vi "FTW-JSON-Interpret-Core.vi"(5 "JSON String":string, 7 "JSON Parent":T1, 9 "Starting Offset":i32, 11 "error in":errorcluster) -> (4 "Data Name":string, 6 "JSON Part":T1, 8 "Container":variant, 10 "Offset after Match":i32, 14 "Found Match?":bool, 15 "error out":errorcluster)   [LabVIEW 2015]
uses:
  FTW-JSON-Part.ctl
panel:
  out "Match":string
  # "Inputs"
  # "Outputs"
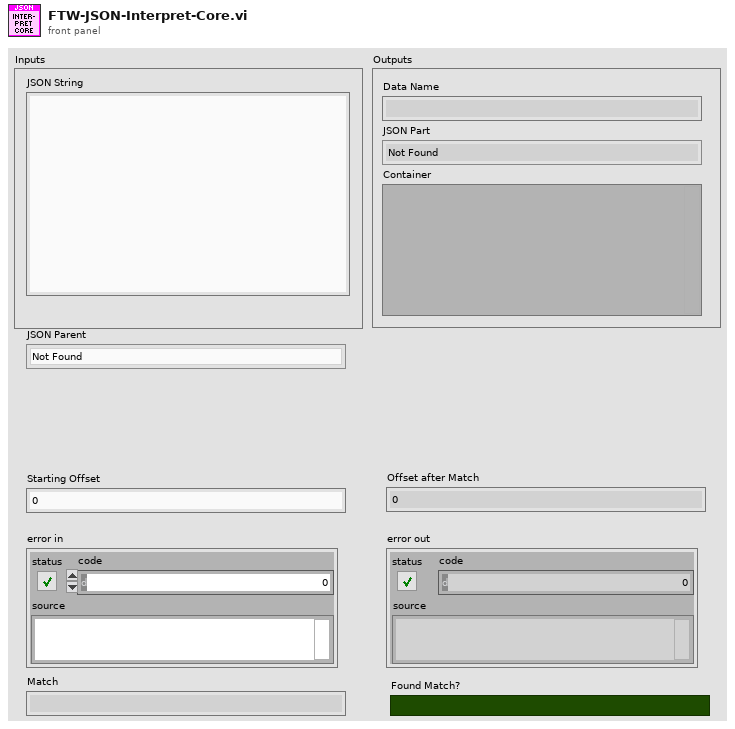
[diagram p1: front panel]
types:
  T1 = typedef "FTW-JSON-Part.ctl" = enum8{"Not Found", "Object", "Object Inner", "Array", "Array Inner", "String", "Number", "Boolean", "null"}
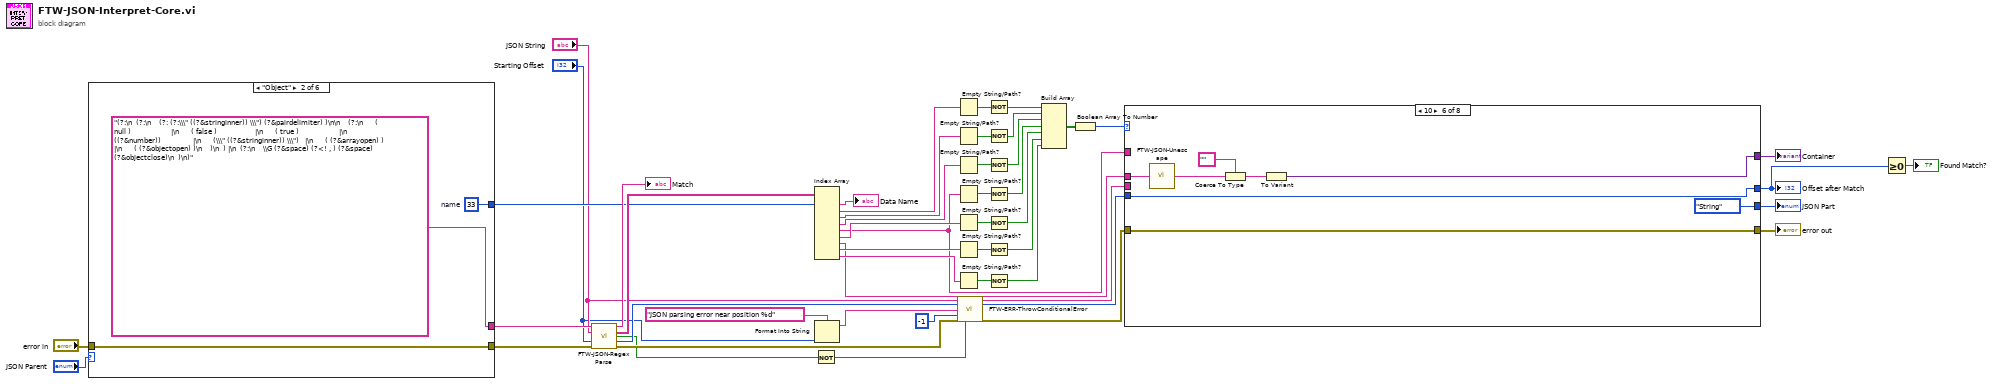
[diagram p0: block diagram]
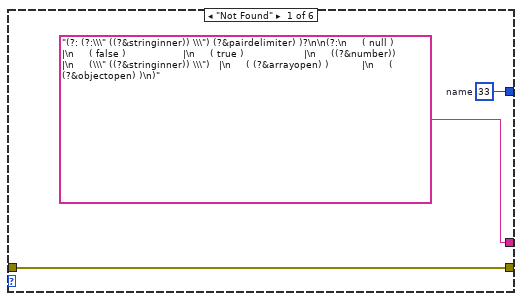
[diagram p2: hidden frame]
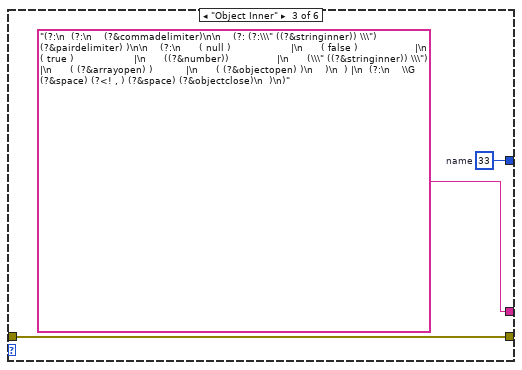
[diagram p3: hidden frame]
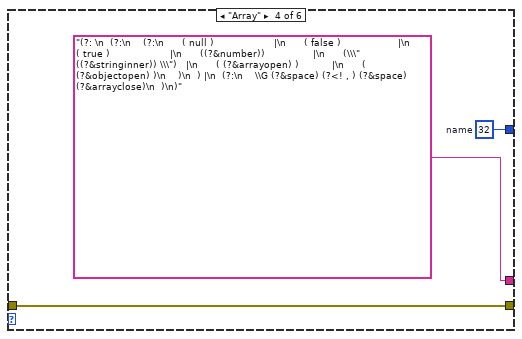
[diagram p4: hidden frame]
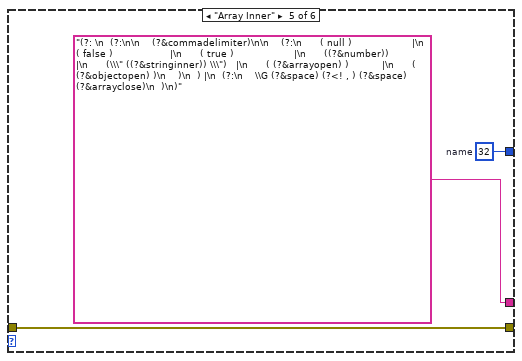
[diagram p5: hidden frame]
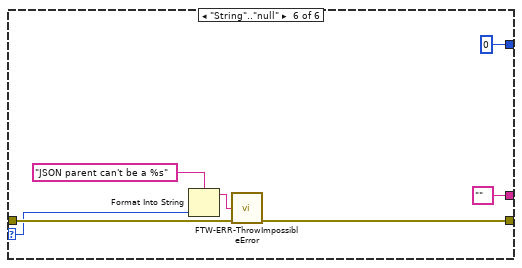
[diagram p6: hidden frame]
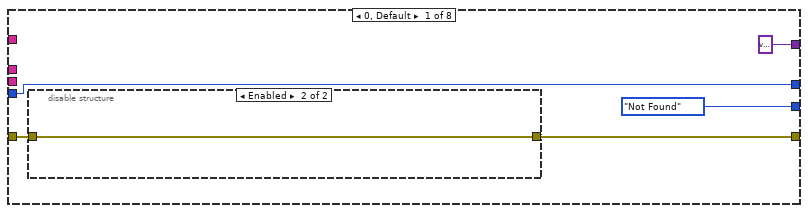
[diagram p7: hidden frame]
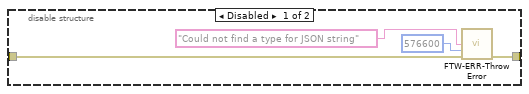
[diagram p8: hidden frame]
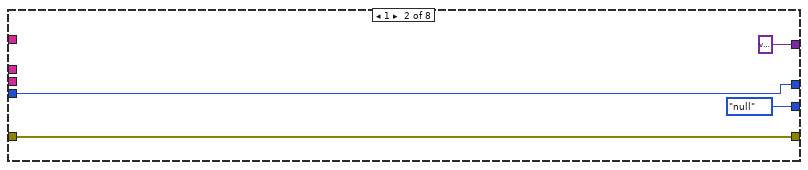
[diagram p9: hidden frame]
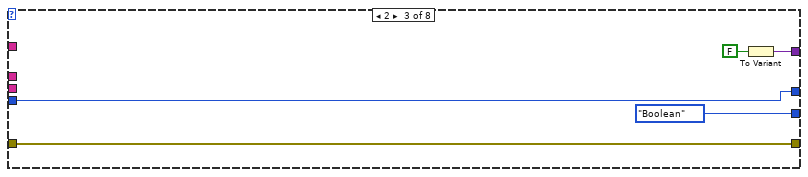
[diagram p10: hidden frame]
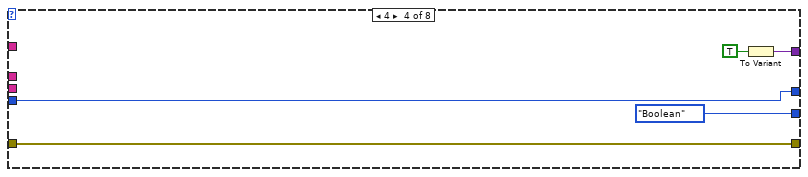
[diagram p11: hidden frame]
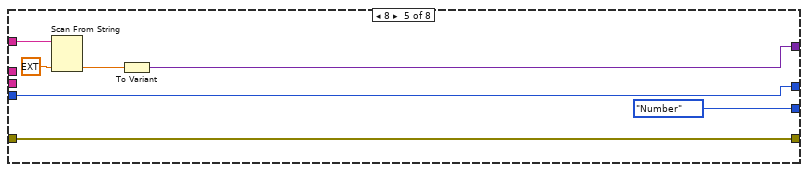
[diagram p12: hidden frame]
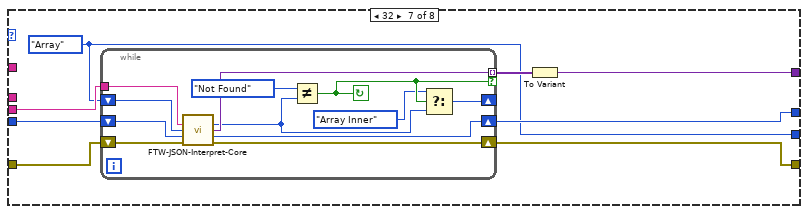
[diagram p13: hidden frame]
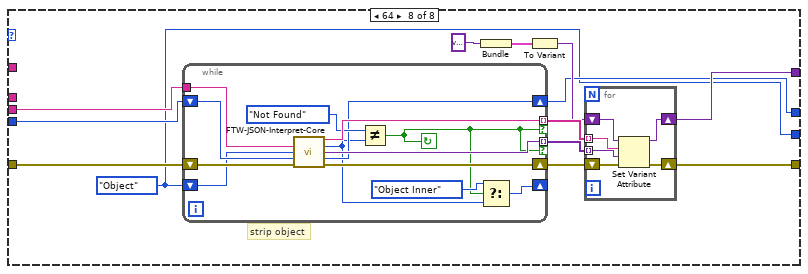
[diagram p14: hidden frame]
diagram:
  n1 = case shown="\"Object\"" "JSON Parent" {
    selector: "JSON Parent" -> [_ _ _ _ _ w66]
    tunnel: ["(?: (?:\\\" ((?&stringinner)) \\\") (?&pairdelimiter) )?\n\n(?:\n     ( null )                    |\n     ( false )                   |\n     ( true )                    |\n     ((?&number))                |\n     (\\\" ((?&stringinner)) \\\")   |\n     ( (?&arrayopen) )           |\n     ( (?&objectopen) )\n)" "(?:\n  (?:\n    (?: (?:\\\" ((?&stringinner)) \\\") (?&pairdelimiter) )\n\n    (?:\n      ( null )                    |\n      ( false )                   |\n      ( true )                    |\n      ((?&number))                |\n      (\\\" ((?&stringinner)) \\\")   |\n      ( (?&arrayopen) )           |\n      ( (?&objectopen) )\n    )\n  ) |\n  (?:\n    \\G (?&space) (?<! , ) (?&space) (?&objectclose)\n  )\n)" "(?:\n  (?:\n    (?&commadelimiter)\n\n    (?: (?:\\\" ((?&stringinner)) \\\") (?&pairdelimiter) )\n\n    (?:\n      ( null )                    |\n      ( false )                   |\n      ( true )                    |\n      ((?&number))                |\n      (\\\" ((?&stringinner)) \\\")   |\n      ( (?&arrayopen) )           |\n      ( (?&objectopen) )\n    )\n  ) |\n  (?:\n    \\G (?&space) (?<! , ) (?&space) (?&objectclose)\n  )\n)" "(?: \n  (?:\n    (?:\n      ( null )                    |\n      ( false )                   |\n      ( true )                    |\n      ((?&number))                |\n      (\\\" ((?&stringinner)) \\\")   |\n      ( (?&arrayopen) )           |\n      ( (?&objectopen) )\n    )\n  ) |\n  (?:\n    \\G (?&space) (?<! , ) (?&space) (?&arrayclose)\n  )\n)" "(?: \n  (?:\n\n    (?&commadelimiter)\n\n    (?:\n      ( null )                    |\n      ( false )                   |\n      ( true )                    |\n      ((?&number))                |\n      (\\\" ((?&stringinner)) \\\")   |\n      ( (?&arrayopen) )           |\n      ( (?&objectopen) )\n    )\n  ) |\n  (?:\n    \\G (?&space) (?<! , ) (?&space) (?&arrayclose)\n  )\n)" "" ("empty string")] -> w13
    tunnel: [w49 w52 w55 w58 w61 w68] -> w20
    tunnel: "error in" -> [w49 w52 w55 w58 w61 w69]
    tunnel: [w48 w51 w54 w57 w60 0] -> w18
    frame "Not Found" {
      w48 = 33  # name
    }
    frame "Object" {
      w51 = 33  # name
    }
    frame "Object Inner" {
      w54 = 33  # name
    }
    frame "Array" {
      w57 = 32  # name
    }
    frame "Array Inner" {
      w60 = 32  # name
    }
    frame "String".."null" {
      n2 = Format Into String(format string="JSON parent can't be a %s" ("Reason this error should never happen"), w66) -> (resulting string=w65:string)  [unwired: 2 in, 1 out]
      n3 = call "FTW-ERR-ThrowImpossibleError.vi"("Reason this error should never happen"=w65, "error in"=w69) -> ("error out"=w68:errorcluster)  [unwired: 13 in]
    }
  }
  n4 = call "FTW-JSON-RegexParse.vi"("Regular Expression using JSON subroutines"=w13, "Input String"="JSON String", "Starting Offset"="Starting Offset", "error in"=w20) -> ("Match"=→"Match":string, "Submatches"=w40:string[], "Found Match?"=w8:bool, "Offset after Match"=w12:i32, "error out"=w43:errorcluster)  [unwired: 7 in]
  n5 = Not(x=w8) -> (.not. x?=w7:bool)
  n6 = Index Array(array=w40, index #1=w18) -> (element #1=→"Data Name":string, element #2=w41:string, element #3=w34:string, element #4=w28:string, element #5=w11:string, element #6=w15:string, element #7=w14:string, element #8=w17:string, element #9=w16:string)  [unwired: 8 in]
  n7 = Format Into String(format string="JSON parsing error near position %d", "Starting Offset") -> (resulting string=w4:string)  [unwired: 2 in, 1 out]
  n8 = Empty String/Path?(string/path=w41) -> (empty?=w39:bool)
  n9 = Empty String/Path?(string/path=w34) -> (empty?=w35:bool)
  n10 = Empty String/Path?(string/path=w28) -> (empty?=w32:bool)
  n11 = Empty String/Path?(string/path=w11) -> (empty?=w31:bool)
  n12 = Empty String/Path?(string/path=w15) -> (empty?=w27:bool)
  n13 = Empty String/Path?(string/path=w17) -> (empty?=w24:bool)
  n14 = Empty String/Path?(string/path=w16) -> (empty?=w25:bool)
  n15 = call "FTW-ERR-ThrowConditionalError.vi"("Error Message"=w4, "Error Code"=-1, "error in"=w43, "Throw Error?"=w7) -> ("error out"=w9:errorcluster)  [unwired: 11 in]
  n16 = Not(x=w39) -> (.not. x?=w38:bool)
  n17 = Not(x=w35) -> (.not. x?=w33:bool)
  n18 = Not(x=w32) -> (.not. x?=w30:bool)
  n19 = Not(x=w31) -> (.not. x?=w29:bool)
  n20 = Not(x=w27) -> (.not. x?=w26:bool)
  n21 = Not(x=w24) -> (.not. x?=w23:bool)
  n22 = Not(x=w25) -> (.not. x?=w22:bool)
  n23 = Build Array(w38, w33, w30, w29, w26, w23, w22) -> (w37:bool[])
  n24 = Boolean Array To Number(Boolean array=w37) -> (number=w36:u32)
  n25 = case shown="10" w36 {
    tunnel: [FTW-JSON-Part."Not Found" ("JSON Type") FTW-JSON-Part."null" ("JSON Type") FTW-JSON-Part."Boolean" ("JSON Type") FTW-JSON-Part."Boolean" ("JSON Type") FTW-JSON-Part."Number" ("JSON Type") FTW-JSON-Part."String" ("JSON Type") w109 w129] -> w45
    tunnel: [variant variant w87 w92 w98 w107 w116 w141] -> w44
    tunnel: w9 -> [w72 w81 w86 w91 w96 w106 w115 w140]
    tunnel: [w71 w81 w86 w91 w96 w106 w114 w139] -> w42
    tunnel: w11 -> [_ _ _ _ w95 _ _ _]
    tunnel: w14 -> [_ _ _ _ _ w104 _ _]
    tunnel: "JSON String" -> [_ _ _ _ _ _ w112 w131]
    tunnel: w12 -> [w70 w80 w84 w89 w94 w103 w111 w132]
    tunnel: [w70 w80 w84 w89 w94 w103 w110 w130] -> w2
    frame 0, Default {
      n26 = disable-structure shown="Enabled" {
        disable-tunnel: w72 -> [w78 w79]
        disable-tunnel: [w77 w79] -> w71
        frame Disabled {
          n27 = call "FTW-ERR-ThrowError.vi"("Error Message"="Could not find a type for JSON string", "Error Code"=576600, "error in"=w78) -> ("error out"=w77:errorcluster)  [unwired: 12 in]
        }
        frame Enabled {
        }
      }
    }
    frame 1 {
    }
    frame 2 {
      n28 = To Variant(anything=FALSE) -> (Variant=w87:variant)
    }
    frame 4 {
      n29 = To Variant(anything=TRUE) -> (Variant=w92:variant)
    }
    frame 8 {
      n30 = Scan From String(input string=w95, default 1=ext 0.0) -> (output 1=w99:ext)  [unwired: 3 in, 3 out]
      n31 = To Variant(anything=w99) -> (Variant=w98:variant)
    }
    frame 16 {
      n32 = call "FTW-JSON-Unescape.vi"("Escaped UTF-8 String"=w104) -> ("Unescaped String"=w101:string)
      n33 = Coerce To Type(0:w101, 1:"") -> (2:w102:string)
      n34 = To Variant(anything=w102) -> (Variant=w107:variant)
    }
    frame 32 {
      w109 = FTW-JSON-Part."Array" ("JSON Type")
      n35 = while {
        tunnel: w112 -> [w128]
        tunnel: [w127] -> w113 mode=indexing if=w118
        shift-right: [w124] -> w110
        shift-left: w111 -> [w125]
        shift-right: [w122] -> w114
        shift-left: w115 -> [w123]
        shift-right: [w119] -> _
        shift-left: w109 -> [w121]
        stop <- w118 continue-if-true
        n36 = call "FTW-JSON-Interpret-Core.vi"("JSON String"=w128, "JSON Parent"=w121, "Starting Offset"=w125, "error in"=w123) -> ("JSON Part"=w120:T1, "Container"=w127:variant, "Offset after Match"=w124:i32, "error out"=w122:errorcluster)  [unwired: 6 in, 2 out]
        n37 = Not Equal?(x=FTW-JSON-Part."Not Found" ("y"), y=w120) -> (x != y?=w118:bool)
        n38 = Select(t=FTW-JSON-Part."Array Inner", s=w118, f=w120) -> (s? t:f=w119:T1)
      }
      n39 = To Variant(anything=w113) -> (Variant=w116:variant)
    }
    frame 64 {
      w129 = FTW-JSON-Part."Object" ("JSON Type")
      # "strip object"
      n40 = while {
        tunnel: w131 -> [w160]
        tunnel: [w159] -> w137 mode=indexing if=w148
        tunnel: [w158] -> w136 mode=indexing if=w148
        shift-right: [w155] -> w130
        shift-left: w132 -> [w156]
        shift-right: [w153] -> w135
        shift-left: w140 -> [w154]
        shift-right: [w149] -> _
        shift-left: w129 -> [w152]
        stop <- w148 continue-if-true
        n41 = call "FTW-JSON-Interpret-Core.vi"("JSON String"=w160, "JSON Parent"=w152, "Starting Offset"=w156, "error in"=w154) -> ("Data Name"=w159:string, "JSON Part"=w150:T1, "Container"=w158:variant, "Offset after Match"=w155:i32, "error out"=w153:errorcluster)  [unwired: 6 in, 1 out]
        n42 = Not Equal?(x=FTW-JSON-Part."Not Found" ("y"), y=w150) -> (x != y?=w148:bool)
        n43 = Select(t=FTW-JSON-Part."Object Inner", s=w148, f=w150) -> (s? t:f=w149:T1)
      }
      n44 = Bundle(variant) -> (w134:cluster{variant})  [unwired: 1 in]
      n45 = To Variant(anything=w134) -> (Variant=w133:variant)
      n46 = for {
        shift-right: [w146] -> w141
        shift-left: w133 -> [w147]
        tunnel: w137 -> [w145] mode=indexing
        tunnel: w136 -> [w144] mode=indexing
        shift-right: [w142] -> w139
        shift-left: w135 -> [w143]
        n47 = Set Variant Attribute(Variant=w147, name=w145, value=w144, error in=w143) -> (Variant out=w146:variant, error out=w142:errorcluster)  [unwired: 1 out]
      }
    }
  }
  "JSON Part" <- w45
  "Container" <- w44
  "error out" <- w42
  "Offset after Match" <- w2
  n48 = Greater Or Equal To 0?(x=w2) -> (x >= 0?=→"Found Match?":bool)
